vi "Write File interpreter.lvclass.vi"(8 "error in (no error)":errorcluster, 10 "File interpreter.lvclass":refnum<class "File interpreter.lvclass">, 11 "AutoExp in":refnum<class "AutoExp.lvclass">) -> (0 "error out":errorcluster, 3 "AutoExp out":refnum<class "AutoExp.lvclass">)   [LabVIEW 2018]
uses:
  AutoExp.lvclass
  File interpreter/File interpreter.lvclass
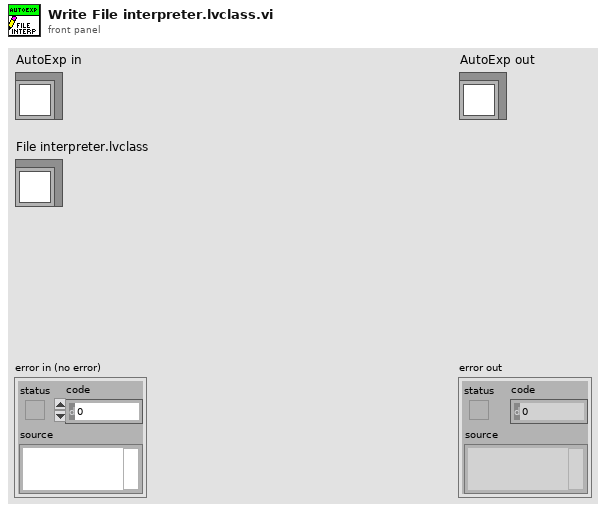
[diagram p1: front panel]
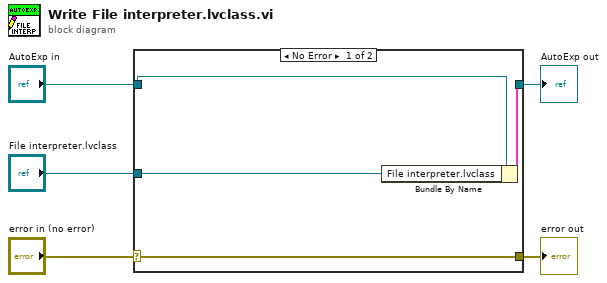
[diagram p0: block diagram]
diagram:
  n1 = case shown="No Error" "error in (no error)" {
    selector: "error in (no error)" -> [w9 w10]
    tunnel: [w9 w10] -> w4
    tunnel: [w7 w11] -> w2
    tunnel: "AutoExp in" -> [w8 w11]
    tunnel: "File interpreter.lvclass" -> [w6 _]
    frame No Error {
      n2 = Bundle By Name(cluster=w8, "File interpreter.lvclass"=w6) -> (w7:cluster{})
    }
    frame Error {
    }
  }
  "error out" <- w4
  "AutoExp out" <- w2
